vi "Set Symbols.vi"(8 "error in (no error)":errorcluster, 9 "Symbols":map{string, string}(c390), 10 "Project Path":path, 11 "App Instance":refnum<vi>) -> (0 "error out":errorcluster)   [LabVIEW 2020, in "Conditional Disabled Configurator.lvclass"]
uses:
  Conditional Disabled Configurator.lvclass
  Conditional Disabled Configurator.lvclass/Conditional Disabled Configurator.ctl
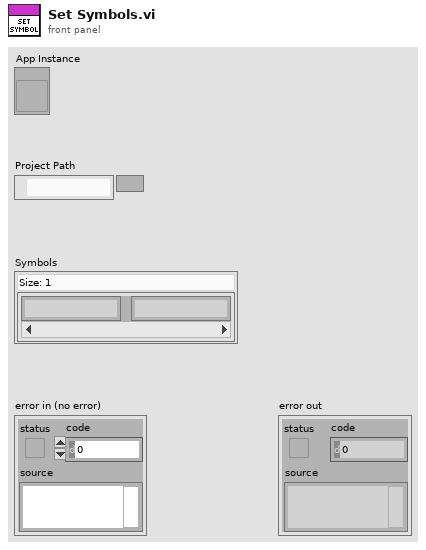
[diagram p1: front panel]
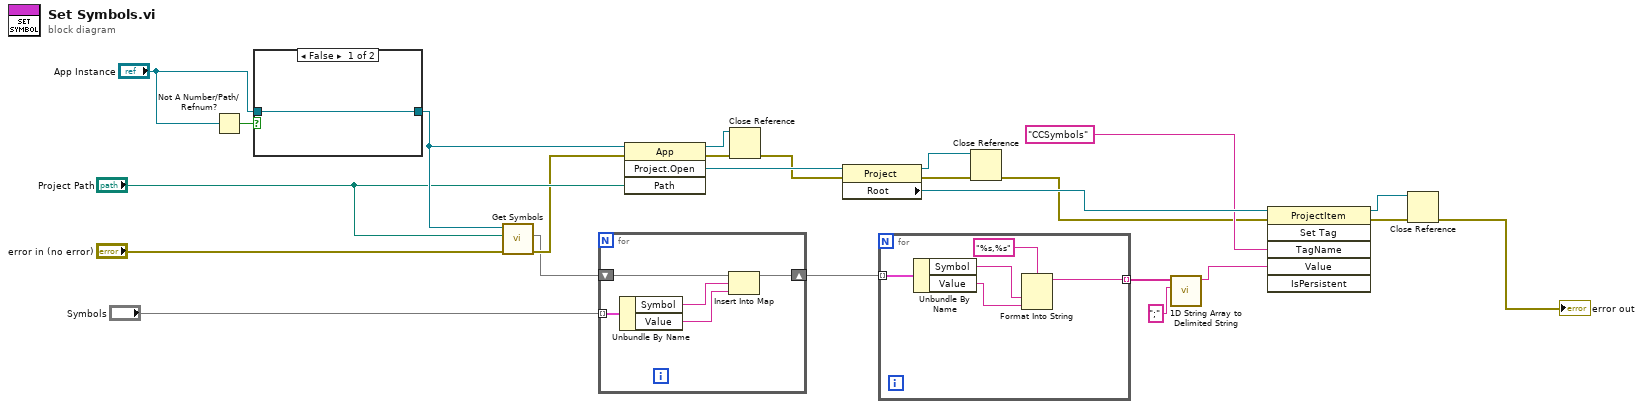
[diagram p0: block diagram]
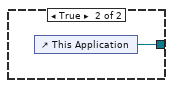
[diagram p2: hidden frame]
diagram:
  n1 = Not A Number/Path/Refnum?(number/path/refnum="App Instance") -> (NaN/Path/Refnum?=w19:bool)
  n2 = case shown="False" w19 {
    tunnel: [w25 w26] -> w17
    tunnel: "App Instance" -> [w25 _]
    frame False {
    }
    frame True {
      n3 = control-ref of="This Application"() -> (w26:refnum<vi>)
    }
  }
  n4 = call "Get Symbols.vi"("error in (no error)"="error in (no error)", "Project Path"="Project Path", "App Instance"=w17) -> ("error out"=w14:errorcluster, "Symbols"=w13:map{string, string})  [unwired: 7 in]
  n5 = for {
    shift-right: [w30] -> w11
    shift-left: w13 -> [w31]
    tunnel: "Symbols" -> [w29] mode=indexing
    n6 = Unbundle By Name(w29) -> ("Symbol"=w28:string, "Value"=w27:string)
    n7 = Insert Into Map(map in=w31, key=w28, value=w27) -> (map out=w30:map{string, string})  [unwired: 2 out]
  }
  n8 = invoke class="App" method="Project.Open"(reference=w17, error in=w14, "Path"="Project Path") -> (reference out=w1:refnum<vi>, error out=w21:errorcluster, "Project:Open"=w24:refnum<vi>)  [unwired: 1 in, 1 out]
  n9 = Close Reference(reference=w1, error in (no error)=w21) -> (error out=w2:errorcluster)
  n10 = property class="Project"(reference=w24, error in=w2) -> (reference out=w3:refnum<vi>, error out=w20:errorcluster, "Root"=w23:refnum<vi>)
  n11 = for {
    tunnel: w11 -> [w36] mode=indexing
    tunnel: [w32] -> w10 mode=indexing
    n12 = Unbundle By Name(w36) -> ("Symbol"=w34:string, "Value"=w33:string)
    n13 = Format Into String(format string="%s,%s", w34, w33) -> (resulting string=w32:string)  [unwired: 2 in, 1 out]
  }
  n14 = Close Reference(reference=w3, error in (no error)=w20) -> (error out=w4:errorcluster)
  n15 = call <vilib>:"1D String Array to Delimited String.vi"("delimiter"=";", "string array"=w10) -> ("delimited string"=w8:string)  [unwired: 9 in]
  n16 = invoke class="ProjectItem" method="Set Tag"(reference=w23, error in=w4, "TagName"="CCSymbols" ("Tag Name"), "Value"=w8) -> (reference out=w5:refnum<vi>, error out=w7:errorcluster)  [unwired: 2 in, 4 out]
  n17 = Close Reference(reference=w5, error in (no error)=w7) -> (error out=→"error out":errorcluster)
